vi "ReadEmbedded.vi"(6 "timeout in ms (-1)":i32, 8 "error in (no error)":errorcluster, 11 "MAUI in":refnum<class "MAUI.lvclass">) -> (0 "error out":errorcluster, 2 "Subpanels":refnum<class "EmbeddedSMO.lvclass">[](array[class]), 3 "MAUI out":refnum<class "MAUI.lvclass">)   [LabVIEW 2016, in "MAUI.lvclass"]
uses:
  MAUI.lvclass
  <vilib>/Levylab/Embedded SMO UI/EmbeddedSMO.lvclass
  Typedefs/PrivateEvents--MAUI.GetEmbedded.ctl
  MAUI.lvclass/MAUI.ctl
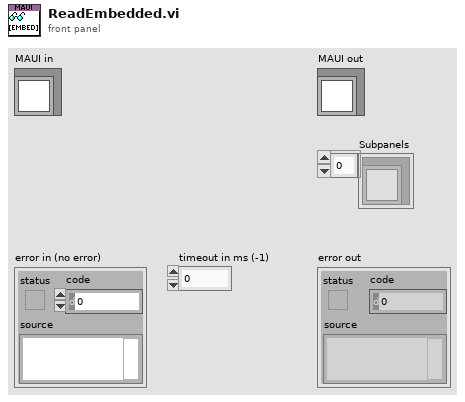
[diagram p1: front panel]
types:
  T1 = typedef "MAUI.lvclass/PrivateEvents--MAUI.GetEmbedded.ctl" = cluster{"notifier out":refnum<notifier>}
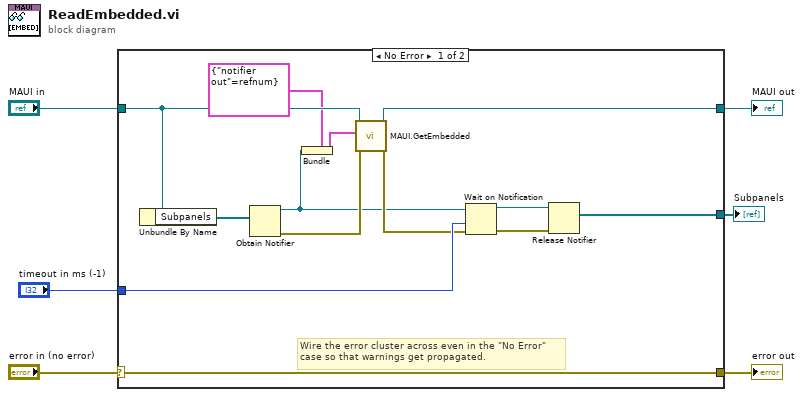
[diagram p0: block diagram]
diagram:
  n1 = case shown="No Error" "error in (no error)" {
    selector: "error in (no error)" -> [w19 w21]
    tunnel: [w19 w21] -> w4
    tunnel: [w12 w20] -> w5
    tunnel: "MAUI in" -> [w13 w20]
    tunnel: "timeout in ms (-1)" -> [w17 _]
    tunnel: [w14 _] -> w1
    frame No Error {
      # "Wire the error cluster across even in the \"No Error\"\ncase so that warnings get propagated."
      n2 = Unbundle By Name(w13) -> ("Subpanels"=w18:refnum<class "EmbeddedSMO.lvclass">[])
      n3 = Obtain Notifier(notification data type=w18) -> (notifier out=w7:refnum<notifier>, error out=w11:errorcluster)  [unwired: 3 in, 1 out]
      n4 = Bundle(cluster=T1 {"notifier out"=refnum} ("GetEmbedded"), "notifier out"=w7) -> (w8:T1)
      n5 = call "MAUI.GetEmbedded.vi"("error in (no error)"=w11, "GetEmbedded"=w8, "MAUI"=w13) -> ("error out"=w10:errorcluster, "MAUI out"=w12:refnum<class "MAUI.lvclass">)  [unwired: 7 in]
      n6 = Wait on Notification(notifier=w7, timeout in ms (-1)=w17, error in (no error)=w10) -> (notifier out=w16:refnum<notifier>, error out=w15:errorcluster)  [unwired: 1 in, 2 out]
      n7 = Release Notifier(notifier=w16, error in (no error)=w15) -> (last notification=w14:refnum<class "EmbeddedSMO.lvclass">[])  [unwired: 1 in, 2 out]
    }
    frame Error {
    }
  }
  "error out" <- w4
  "MAUI out" <- w5
  "Subpanels" <- w1
